vi "Read Dispense Parameters.vi"(8 "error in (no error)":errorcluster, 11 "VISA resource name":refnum<visa-resource-name>) -> (0 "error out":errorcluster, 1 "Pressure":dbl, 2 "Dispense Time":dbl, 3 "VISA resource name out":refnum<visa-resource-name>, 5 "Memory Location":i32)   [LabVIEW 2020, in "EFD Ultimus V.lvlib"]
doc: "Reads the Ultimus V's current memory channel, dispense time and dispense pressure to the host. 'D0' is the number zero (0). Modifications need to be made if not using inH20 for vacuum units and psi for pressure units. \n\nHost Format: UD---\n\nReturn Format: D0ChcccPDppppDTtttt\nccc: The 3 digit memory location from 0-511. The dispenser will automatically limit value to prevent any errors.\npppp: The four digit pressure setting. This is a unit less value. The valid pressure ranges and decimal point are determined by the pressure units currently selected in the dispenser. \nttttt: The four digit dispense time. The valid range is 0.000 to 9.999. This command truncates the last decimal place of the dispense time."
uses:
  EFD Ultimus V.lvlib
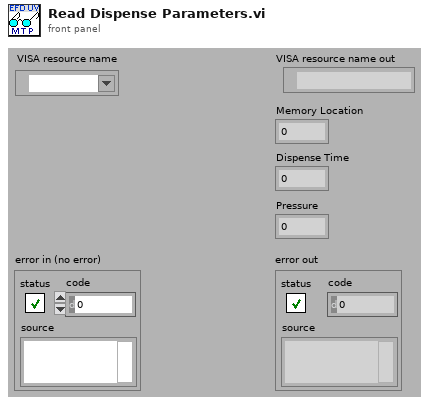
[diagram p1: front panel]
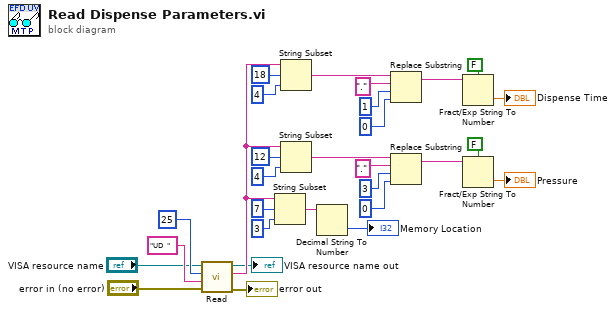
[diagram p0: block diagram]
diagram:
  n1 = call "Read.vi"("error in (no error)"="error in (no error)", "Command To Write"="UD  ", "Bytes to Read (11)"=u32 25 ("Bytes to Read from Buffer"), "VISA resource name"="VISA resource name") -> ("error out"=→"error out":errorcluster, "Ultimus V Feedback Data"=w23:string, "VISA resource name out"=→"VISA resource name out":refnum<visa-resource-name>)  [unwired: 5 out]
  n2 = String Subset(string=w23, offset (0)=7, length (rest)=3 ("length (rest)")) -> (substring=w6:string)
  n3 = String Subset(string=w23, offset (0)=18, length (rest)=4 ("length (rest)")) -> (substring=w18:string)
  n4 = String Subset(string=w23, offset (0)=12, length (rest)=4 ("length (rest)")) -> (substring=w7:string)
  n5 = Decimal String To Number(string=w6) -> (number=→"Memory Location":i32)  [unwired: 3 out]
  n6 = Replace Substring(2:0 ("length (len. of substring)"), 3:1 ("offset (0)"), 4:"." ("substring (\"\")"), 5:w18) -> (1:w14:string)  [unwired: 1 out]
  n7 = Replace Substring(2:0 ("length (len. of substring)"), 3:3 ("offset (0)"), 4:"." ("substring (\"\")"), 5:w7) -> (1:w11:string)  [unwired: 1 out]
  n8 = Fract/Exp String To Number(use system decimal point (T)=FALSE, string=w14) -> (number=→"Dispense Time":dbl)  [unwired: 3 out]
  n9 = Fract/Exp String To Number(use system decimal point (T)=FALSE, string=w11) -> (number=→"Pressure":dbl)  [unwired: 3 out]
